vi "ecc register segment n2e.vi"(1 "number":u8 format="%0d") -> (0 "enum":T1)   [LabVIEW 2024, in "atsj peakcan basic.lvlib"]
uses:
  ecc register segment.ctl
  atsj peakcan basic.lvlib
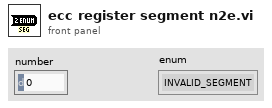
[diagram p1: front panel]
types:
  T1 = typedef "atsj peakcan basic.lvlib/ecc register segment.ctl" = enum8{"INVALID_SEGMENT", "ID_28_TO_ID_21", "START_OF_FRAME", "BIT_SRTR", "BIT_IDE", "ID_20_TO_ID_18", "ID_17_TO_ID_13", "CRC_SEQUENCE", "RESERVED_BIT_0", "DATA_FIELD", "DATA_LENGTH_CODE", "BIT_RTR", "RESERVED_BIT_1", "ID_4_TO_ID_0", "ID_12_TO_ID_5", "ACTIVE_ERROR_FLAG", "INTERMISSION", "TOLERATE_DOMINANT_BITS", "ERROR_DELIMITER", "CRC_DELIMITER", "ACKNOWLEDGE_SLOT", "END_OF_FRAME", "ACKNOWLEDGE_LIMITER", "OVERLOAD_FLAG"}
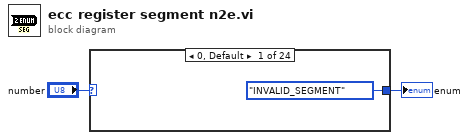
[diagram p0: block diagram]
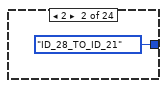
[diagram p2: hidden frame]
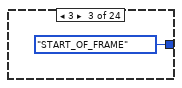
[diagram p3: hidden frame]
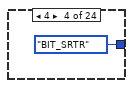
[diagram p4: hidden frame]
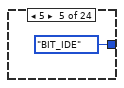
[diagram p5: hidden frame]
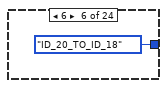
[diagram p6: hidden frame]
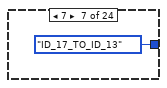
[diagram p7: hidden frame]
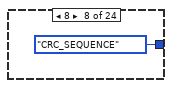
[diagram p8: hidden frame]
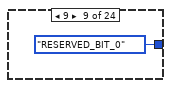
[diagram p9: hidden frame]
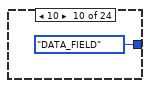
[diagram p10: hidden frame]
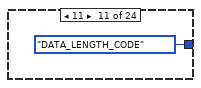
[diagram p11: hidden frame]
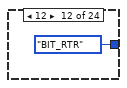
[diagram p12: hidden frame]
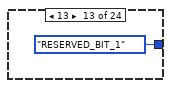
[diagram p13: hidden frame]
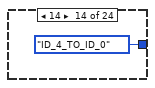
[diagram p14: hidden frame]
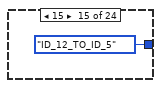
[diagram p15: hidden frame]
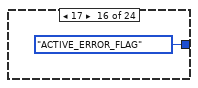
[diagram p16: hidden frame]
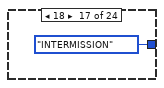
[diagram p17: hidden frame]
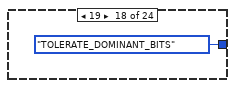
[diagram p18: hidden frame]
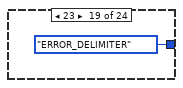
[diagram p19: hidden frame]
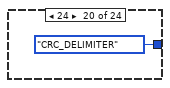
[diagram p20: hidden frame]
diagram:
  n1 = case shown="0, Default" "number" {
    tunnel: [ecc_register_segment."INVALID_SEGMENT" ecc_register_segment."ID_28_TO_ID_21" ecc_register_segment."START_OF_FRAME" ecc_register_segment."BIT_SRTR" ecc_register_segment."BIT_IDE" ecc_register_segment."ID_20_TO_ID_18" ecc_register_segment."ID_17_TO_ID_13" ecc_register_segment."CRC_SEQUENCE" ecc_register_segment."RESERVED_BIT_0" ecc_register_segment."DATA_FIELD" ecc_register_segment."DATA_LENGTH_CODE" ecc_register_segment."BIT_RTR" ecc_register_segment."RESERVED_BIT_1" ecc_register_segment."ID_4_TO_ID_0" ecc_register_segment."ID_12_TO_ID_5" ecc_register_segment."ACTIVE_ERROR_FLAG" ecc_register_segment."INTERMISSION" ecc_register_segment."TOLERATE_DOMINANT_BITS" ecc_register_segment."ERROR_DELIMITER" ecc_register_segment."CRC_DELIMITER" ecc_register_segment."ACKNOWLEDGE_SLOT" ecc_register_segment."END_OF_FRAME" ecc_register_segment."ACKNOWLEDGE_LIMITER" ecc_register_segment."OVERLOAD_FLAG"] -> w1
    frame 0, Default {
    }
    frame 2 {
    }
    frame 3 {
    }
    frame 4 {
    }
    frame 5 {
    }
    frame 6 {
    }
    frame 7 {
    }
    frame 8 {
    }
    frame 9 {
    }
    frame 10 {
    }
    frame 11 {
    }
    frame 12 {
    }
    frame 13 {
    }
    frame 14 {
    }
    frame 15 {
    }
    frame 17 {
    }
    frame 18 {
    }
    frame 19 {
    }
    frame 23 {
    }
    frame 24 {
    }
    frame 25 {
    }
    frame 26 {
    }
    frame 27 {
    }
    frame 28 {
    }
  }
  "enum" <- w1
